vi "S2C_PCIe7841_Proc_ManageSelection.vi"(8 "Error In":errorcluster, 9 "NewValue":variant, 10 "OldValue":variant, 11 "CtlRef":refnum<vi>) -> (0 "Error Out":errorcluster)   [LabVIEW 2015]
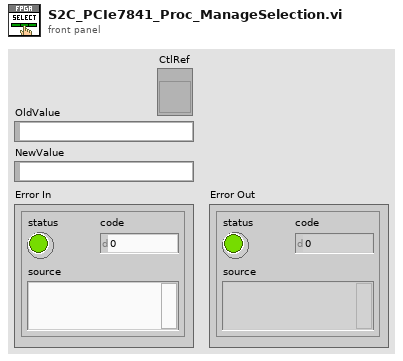
[diagram p1: front panel]
types:
  T1 = cluster{"P0B0":bool, "P0B1":bool, "P0B2":bool, "P0B3":bool, "P0B4":bool, "P0B5":bool, "P0B6":bool, "P0B7":bool, "P0_Send":bool, "P0_Size":bool, "P0_State":bool}
  T2 = cluster{"Port 0[0]":bool, "Port 0[1]":bool, "Port 0[2]":bool, "Port 0[3]":bool, "Port 0[4]":bool, "Port 0[5]":bool, "Port 0[6]":bool, "Port 0[7]":bool, "Port 0[8]":bool, "Port 0[9]":bool, "Port 0[10]":bool}
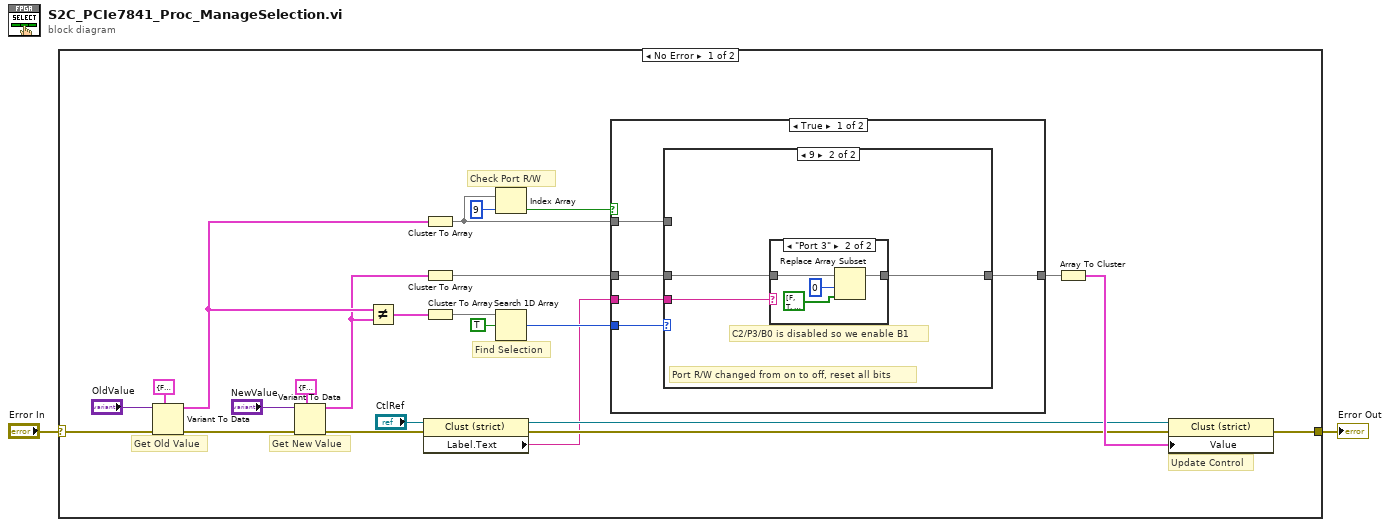
[diagram p0: block diagram]
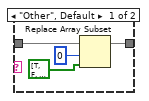
[diagram p3: hidden frame]
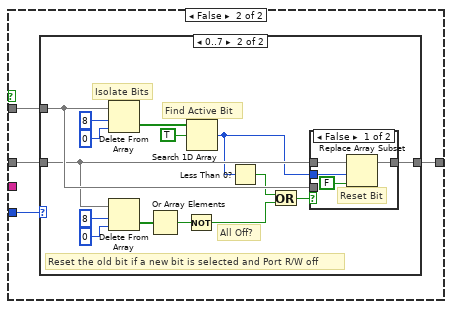
[diagram p4: hidden frame]
diagram:
  n1 = case shown="No Error" "Error In" {
    selector: "Error In" -> [w17 w69]
    tunnel: [w20 w69] -> w1
    frame No Error {
      # "Check Port R/W"
      # "Update Control"
      # "Find Selection"
      # "Get New Value"
      # "Get Old Value"
      n2 = Variant To Data(error in=w17, type=T1 {"P0B0"=FALSE, "P0B1"=TRUE, "P0B2"=FALSE, "P0B3"=FALSE, "P0B4"=FALSE, "P0B5"=FALSE, "P0B6"=FALSE, "P0B7"=FALSE, "P0_Send"=FALSE, "P0_Size"=FALSE, "P0_State"=FALSE} ("Port 0"), Variant="OldValue") -> (data=w13:T1, error out=w16:errorcluster)
      n3 = Variant To Data(error in=w16, type=T1 {"P0B0"=FALSE, "P0B1"=TRUE, "P0B2"=FALSE, "P0B3"=FALSE, "P0B4"=FALSE, "P0B5"=FALSE, "P0B6"=FALSE, "P0B7"=FALSE, "P0_Send"=FALSE, "P0_Size"=FALSE, "P0_State"=FALSE} ("Port 0"), Variant="NewValue") -> (data=w12:T1, error out=w6:errorcluster)
      n4 = Not Equal?(x=w13, y=w12) -> (x != y?=w26:T1)
      n5 = property class="Clust (strict)"(reference="CtlRef", error in=w6) -> (reference out=w4:refnum<vi>, error out=w5:errorcluster, "Label.Text"=w3:string)
      n6 = Cluster To Array(cluster=w13) -> (array=w8:bool[])
      n7 = Cluster To Array(cluster=w12) -> (array=w11:bool[])
      n8 = Cluster To Array(cluster=w26) -> (array=w25:bool[])
      n9 = Index Array(array=w8, index=9) -> (element=w9:bool)
      n10 = Search 1D Array(1D array=w25, element=TRUE) -> (index of element=w24:i32)  [unwired: 1 in]
      n11 = case shown="True" w9 {
        tunnel: w24 -> [w31 w47]
        tunnel: w8 -> [w30 w46]
        tunnel: w11 -> [w29 w45]
        tunnel: [w28 w44] -> w22
        tunnel: w3 -> [w27 _]
        frame True {
          n12 = case shown="9" w31 {
            tunnel: w30 -> [_ _]
            tunnel: w29 -> [w32 w35]
            tunnel: [w32 w34] -> w28
            tunnel: w27 -> [_ w33]
            frame -1, Default {
            }
            frame 9 {
              # "C2/P3/B0 is disabled so we enable B1"
              # "Port R/W changed from on to off, reset all bits"
              n13 = case shown="\"Port 3\"" w33 {
                tunnel: w35 -> [w39 w43]
                tunnel: [w36 w41] -> w34
                frame "Other", Default {
                  n14 = Replace Array Subset(array=w39, new element=bool[] [TRUE, FALSE, FALSE, FALSE, FALSE, FALSE, FALSE, FALSE], index=0) -> (w36:bool[])
                }
                frame "Port 3" {
                  n15 = Replace Array Subset(array=w43, new element=bool[] [FALSE, TRUE, FALSE, FALSE, FALSE, FALSE, FALSE, FALSE], index=0) -> (w41:bool[])
                }
              }
            }
          }
        }
        frame False {
          n16 = case shown="0..7" w47 {
            tunnel: w46 -> [_ w58]
            tunnel: w45 -> [w48 w55]
            tunnel: [w48 w63] -> w44
            frame -1, Default {
            }
            frame 0..7 {
              # "All Off?"
              # "Find Active Bit"
              # "Isolate Bits"
              # "Reset the old bit if a new bit is selected and Port R/W off"
              n17 = Delete From Array(array=w58, length=8, index=0) -> (deleted portion=w60:bool[])  [unwired: 1 out]
              n18 = Delete From Array(array=w55, length=8, index=0) -> (deleted portion=w54:bool[])  [unwired: 1 out]
              n19 = Or Array Elements(Boolean array=w54) -> (logical OR=w51:bool)
              n20 = Not(x=w51) -> (.not. x?=w49:bool)
              n21 = Search 1D Array(1D array=w60, element=TRUE) -> (index of element=w53:i32)  [unwired: 1 in]
              n22 = Less Than 0?(x=w53) -> (x < 0?=w52:bool)
              n23 = Or(x=w52, y=w49) -> (x .or. y?=w50:bool)
              n24 = case shown="False" w50 {
                tunnel: w55 -> [w67 _]
                tunnel: [w66 w68] -> w63
                tunnel: w58 -> [_ w68]
                tunnel: w53 -> [w64 _]
                frame False {
                  # "Reset Bit"
                  n25 = Replace Array Subset(array=w67, new element=FALSE ("new element/subarray"), index=w64) -> (w66:bool[])
                }
                frame True {
                }
              }
            }
          }
        }
      }
      n26 = Array To Cluster(array=w22) -> (cluster=w21:T2)
      n27 = property class="Clust (strict)"(reference=w4, error in=w5, "Value"=w21) -> (error out=w20:errorcluster)  [unwired: 1 out]
    }
    frame Error {
    }
  }
  "Error Out" <- w1
